vi "DataAcquisitionState.vi"(1 "CPU_Overload?":bool, 2 "Above max Temp!":bool, 3 "Temp reached":bool, 4 "Stop?":bool) -> (0 "Channel out":T1)   [LabVIEW 2022 SP3]
uses:
  <extravilib>/ChannelInstances/Stream-str/)Channel.ctl
  <extravilib>/ChannelInstances/Stream-str/Write With Abort.vi
  <extravilib>/ChannelInstances/Stream-str/Endpoint.vi
  <extravilib>/ChannelInstances/Stream-str/)Channel.vi
  <resource>/ChannelSupport/_ChannelSupport/WaitIfNeeded.vi
  <extravilib>/ChannelInstances/Stream-str.lvlib
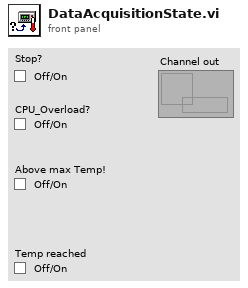
[diagram p1: front panel]
types:
  T1 = typedef "Stream-str.lvlib/)Channel.ctl" = refnum<queue>
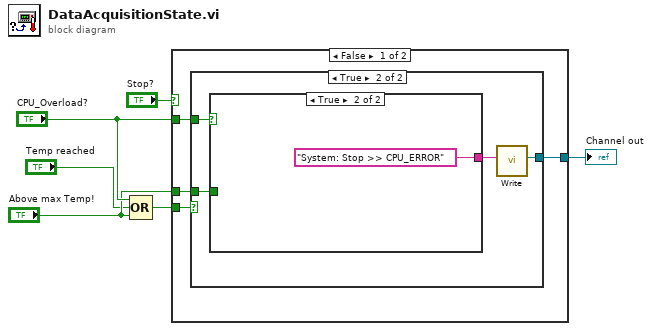
[diagram p0: block diagram]
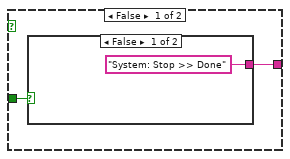
[diagram p3: hidden frame]
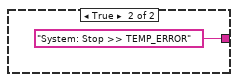
[diagram p4: hidden frame]
diagram:
  n1 = Compound Arithmetic op=OR("CPU_Overload?", "Temp reached", "Above max Temp!") -> (w4:bool)
  n2 = case shown="False" "Stop?" {
    tunnel: "CPU_Overload?" -> [w10 _]
    tunnel: "Above max Temp!" -> [w9 _]
    tunnel: w4 -> [w8 _]
    tunnel: [w7 _] -> w2
    frame False {
      n3 = case shown="True" w8 {
        tunnel: [_ w14] -> w7
        tunnel: w10 -> [_ w13]
        tunnel: w9 -> [_ w11]
        frame False {
        }
        frame True {
          n4 = case shown="True" w13 {
            tunnel: [w15 "System: Stop >> CPU_ERROR" ("t")] -> w12
            tunnel: w11 -> [w16 _]
            frame False {
              n5 = case shown="False" w16 {
                tunnel: ["System: Stop >> Done" "System: Stop >> TEMP_ERROR"] -> w15
                frame False {
                }
                frame True {
                }
              }
            }
            frame True {
            }
          }
          n6 = call <extravilib>:"Write.vi"("element"=w12) -> ("channel"=w14:T1)  [unwired: 8 in, 2 out]
        }
      }
    }
    frame True {
    }
  }
  "Channel out" <- w2
